vi "Seperate Channel Data's.vi"(7 "Data Cluster In":T1, 8 "error In":errorcluster, 11 "RT-Decode Data":T7) -> (0 "error out":errorcluster, 5 "Data Cluster Out":T1)   [LabVIEW 2021, in "Test Panel GUI Update.lvlib"]
uses:
  Test Panel GUI Update.lvlib
  RT-Encode Data.ctl
  Module Data--cluster.ctl
  Test Panel/GUI Ctrl Data's--Cluster.ctl
  Test Panel/Rx-Mapping Data.ctl
  Capsule-Data's.ctl
  Host-Control's/DIO Data's from RT.ctl
  Host-Control's/AI-Data from RT.ctl
  <vilib>/Utility/miscctls.llb/LVMapReplaceAction.ctl
  Test Panel/Test Panel.lvlib
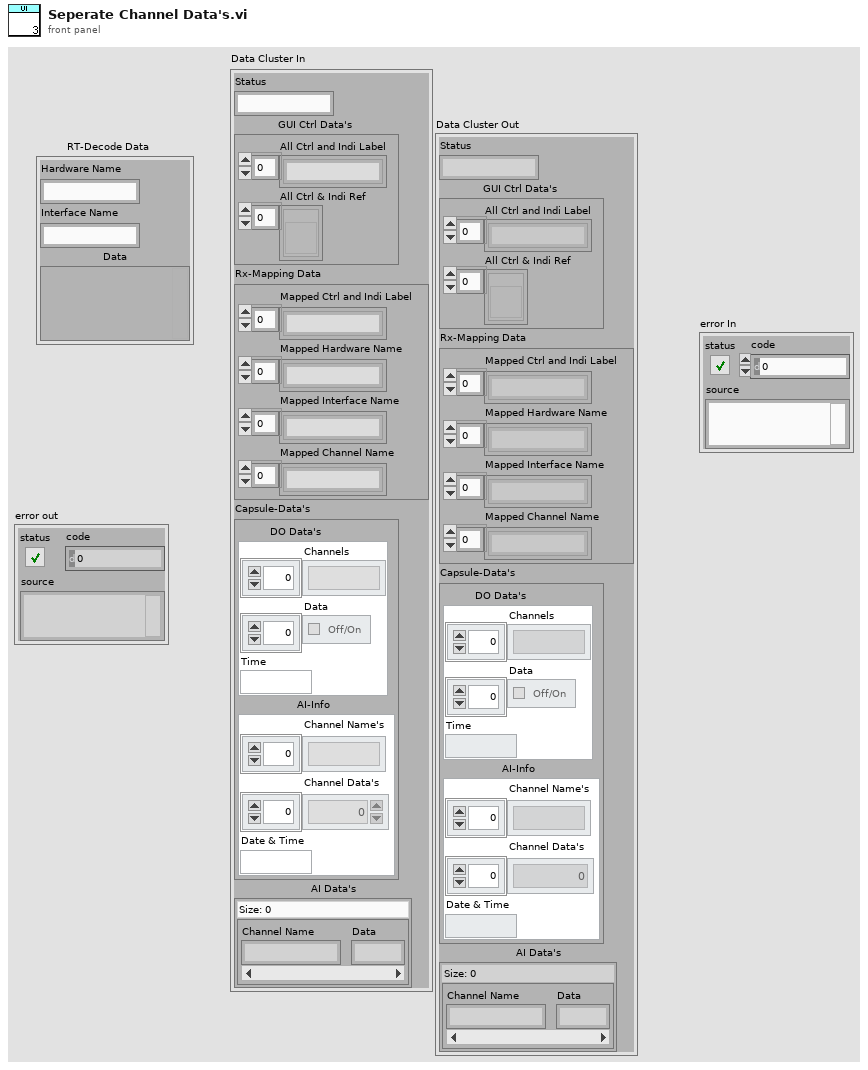
[diagram p1: front panel]
types:
  T1 = typedef "Test Panel GUI Update.lvlib/Module Data--cluster.ctl" = cluster{"Status":string, "GUI Ctrl Data's":T2, "Rx-Mapping Data":T3, "Capsule-Data's":T4, "AI Data's":map{string, dbl}}
  T2 = typedef "Test Panel.lvlib/GUI Ctrl Data's--Cluster.ctl" = cluster{"All Ctrl and Indi Label":string[], "All Ctrl & Indi Ref":refnum<vi>[]}
  T3 = typedef "Test Panel.lvlib/Rx-Mapping Data.ctl" = cluster{"Mapped Ctrl and Indi Label":string[], "Mapped Hardware Name":string[], "Mapped Interface Name":string[], "Mapped Channel Name":string[]}
  T4 = typedef "Test Panel GUI Update.lvlib/Capsule-Data's.ctl" = cluster{"DIO Data's":T5, "AI-Info":T6}
  T5 = typedef "DIO Data's from RT.ctl" = cluster{"Channels":string[], "Data":bool[], "Time":string}
  T6 = typedef "AI-Data from RT.ctl" = cluster{"Channel Name's":string[], "Channel Data's":dbl[], "Date & Time":string}
  T7 = typedef "Test Panel GUI Update.lvlib/RT-Encode Data.ctl" = cluster{"Hardware Name":string, "Interface Name":string, "Data":variant}
  T8 = typedef "LVMapReplaceAction.ctl" = enum32{"Modify Entry only if found", "Add or Modify Entry", "Delete Entry"}
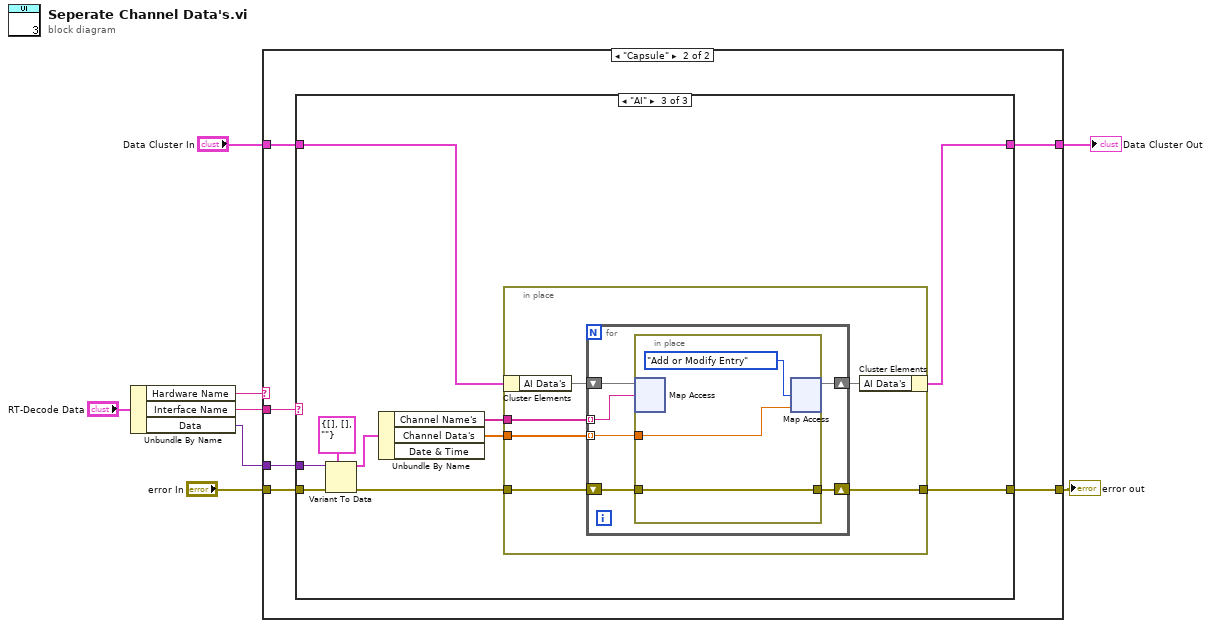
[diagram p0: block diagram]
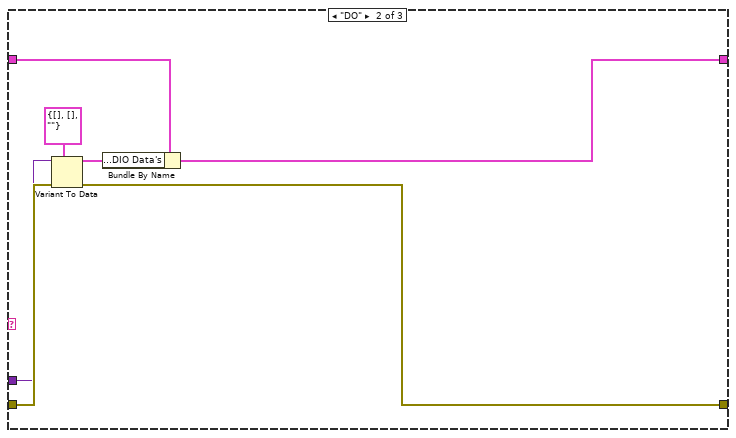
[diagram p4: hidden frame]
diagram:
  n1 = Unbundle By Name("RT-Decode Data") -> ("Hardware Name"=w1:string, "Interface Name"=w2:string, "Data"=w3:variant)
  n2 = case shown="\"Capsule\"" w1 {
    tunnel: w2 -> [_ w14]
    tunnel: w3 -> [_ w15]
    tunnel: "error In" -> [w10 w16]
    tunnel: [w10 w13] -> w6
    tunnel: "Data Cluster In" -> [w9 w12]
    tunnel: [w9 w11] -> w5
    frame "False", Default {
    }
    frame "Capsule" {
      n3 = case shown="\"AI\"" w14 {
        tunnel: w16 -> [w17 w25 w35]
        tunnel: w15 -> [_ w24 w34]
        tunnel: [w17 w23 w29] -> w13
        tunnel: w12 -> [w18 w21 w27]
        tunnel: [w18 w20 w26] -> w11
        frame "False", Default {
        }
        frame "DO" {
          n4 = Variant To Data(error in=w25, type=T5 {"Channels"=[], "Data"=[], "Time"=""} ("DO Data's"), Variant=w24) -> (data=w19:T5, error out=w23:errorcluster)
          n5 = Bundle By Name(cluster=w21, "Capsule-Data's.DIO Data's"=w19) -> (w20:T1)
        }
        frame "AI" {
          n6 = Variant To Data(error in=w35, type=T6 {"Channel Name's"=[], "Channel Data's"=[], "Date & Time"=""} ("AI-Info"), Variant=w34) -> (data=w32:T6, error out=w28:errorcluster)
          n7 = Unbundle By Name(w32) -> ("Channel Name's"=w31:string[], "Channel Data's"=w30:dbl[])  [unwired: 1 out]
          n8 = in-place {
            in-place-border: w31 -> [w41]
            in-place-border: w30 -> [w40]
            in-place-border: [w39] -> w29
            in-place-border: w28 -> [w38]
            n9 = in-place-cluster #1(w27) -> ("AI Data's"=w37:map{string, dbl})
            n10 = for {
              tunnel: w41 -> [w43] mode=indexing
              tunnel: w40 -> [w42] mode=indexing
              shift-right: [w46] -> w39
              shift-left: w38 -> [w47]
              shift-right: [w44] -> w36
              shift-left: w37 -> [w45]
              n11 = in-place {
                in-place-border: w47 -> [w50]
                in-place-border: [w50] -> w46
                in-place-border: w42 -> [w48]
                n12 = in-place-map #2(w45, w43) -> ()  [unwired: 1 in, 2 out]
                n13 = in-place-map #2(w48, LVMapReplaceAction."Add or Modify Entry" ("action")) -> (w44:map{string, dbl})  [unwired: 2 out]
              }
            }
            n14 = in-place-cluster #1("AI Data's"=w36) -> (w26:T1)
          }
        }
      }
    }
  }
  "error out" <- w6
  "Data Cluster Out" <- w5
